vi "RTM - Remove Packet.vi"() -> ()   [LabVIEW 2016, in "UDP-Custom-Device System Explorer.lvlib"]
uses:
  UDP-Custom-Device System Explorer.lvlib
  Shared/Constants.vi
  <vilib>/NI Veristand/Custom Device API/Get Item Property (I32 Array).vi
  <vilib>/NI Veristand/Custom Device API/Get Item Property (String Array).vi
  <vilib>/NI Veristand/Custom Device API/Set Item Property (I32 Array).vi
  <vilib>/NI Veristand/Custom Device API/Set Item Property (String Array).vi
  Shared/UDP-Custom-Device Shared.lvlib
  <vilib>/NI VeriStand/Custom Device API/Custom Device API.lvlib
  <vilib>/NI VeriStand/Custom Device Tools/Custom Device Utility Library/Custom Device Utility Library.lvlib
panel:
  in  "Tag":string
  in  "Node Ptr":u64 format="%.0x"
  out "error out":errorcluster
  in  "error in (no error)":errorcluster
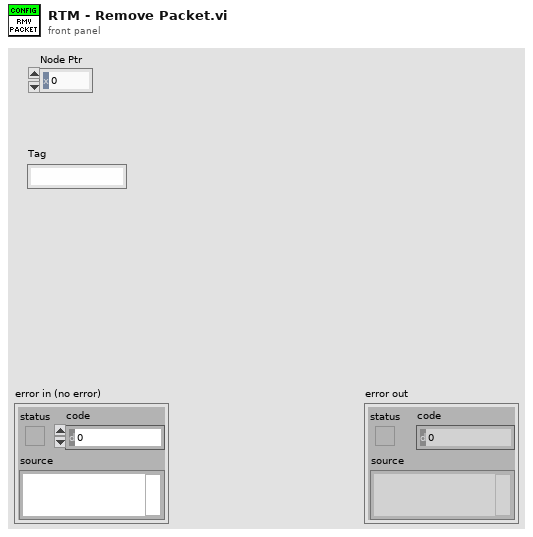
[diagram p1: front panel]
types:
  T1 = typedef "Custom Device API.lvlib/Custom Device Item Ref.ctl" = u64
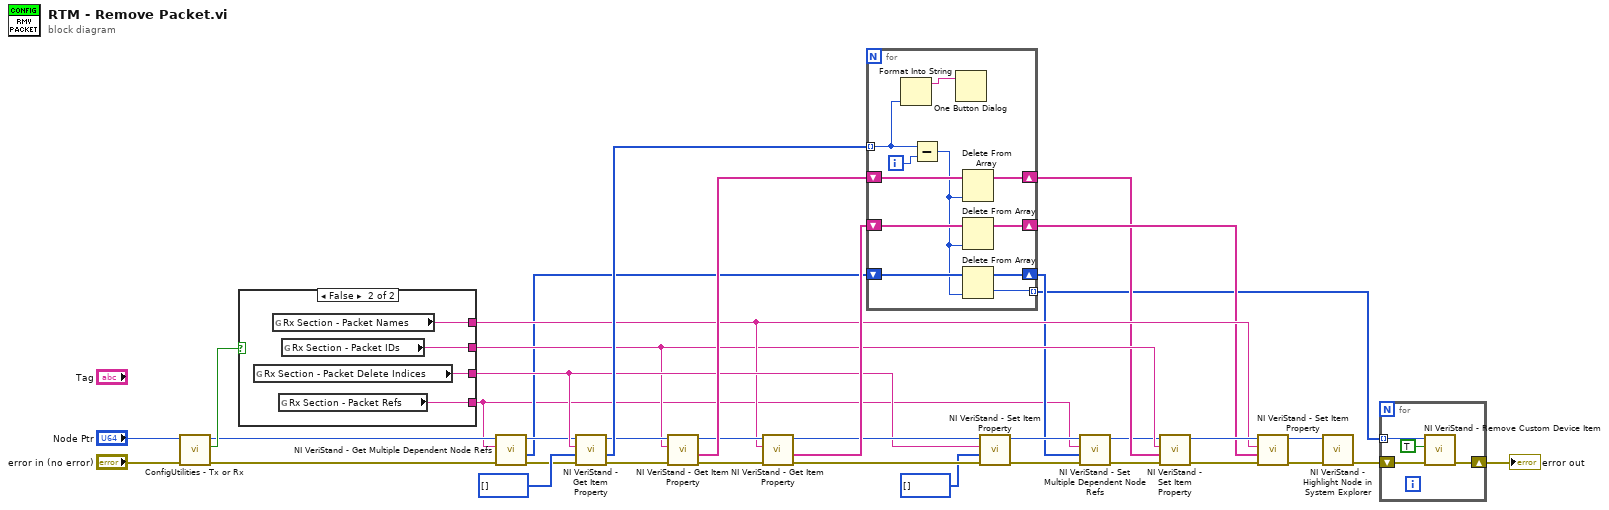
[diagram p0: block diagram]
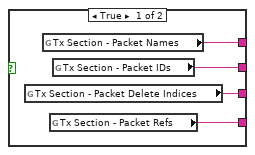
[diagram p2: hidden frame]
diagram:
  n1 = call "ConfigUtilities - Tx or Rx.vi"("error in (no error)"="error in (no error)", "Item Ref in"="Node Ptr") -> ("error out"=w34:errorcluster, "Tx?"=w35:bool, "Item Ref out"=w10:T1)  [unwired: 7 in]
  n2 = case shown="False" w35 {
    tunnel: [w41 w45] -> w19
    tunnel: [w40 w44] -> w18
    tunnel: [w39 w43] -> w23
    tunnel: [w38 w42] -> w3
    frame True {
      n3 = global read "Constants.vi" "Tx Section - Packet Delete Indices"() -> (w39:string)
      n4 = global read "Constants.vi" "Tx Section - Packet Names"() -> (w41:string)
      n5 = global read "Constants.vi" "Tx Section - Packet Refs"() -> (w38:string)
      n6 = global read "Constants.vi" "Tx Section - Packet IDs"() -> (w40:string)
    }
    frame False {
      n7 = global read "Constants.vi" "Rx Section - Packet Delete Indices"() -> (w43:string)
      n8 = global read "Constants.vi" "Rx Section - Packet Names"() -> (w45:string)
      n9 = global read "Constants.vi" "Rx Section - Packet Refs"() -> (w42:string)
      n10 = global read "Constants.vi" "Rx Section - Packet IDs"() -> (w44:string)
    }
  }
  n11 = call <vilib>:"NI VeriStand - Get Multiple Dependent Node Refs.vi"("error in (no error)"=w34, "Base Property Name"=w3, "Item Ref in"=w10) -> ("error out"=w11:errorcluster, "Dependent Node Refs"=w8:T1[], "Item Ref out"=w9:T1)  [unwired: 6 in]
  n12 = call-poly <vilib>:"NI VeriStand - Get Item Property.vi"("error in (no error)"=w11, "Default Value"=i32[] [], "Property Name"=w23, "Item Ref in"=w9) -> ("error out"=w30:errorcluster, "Value"=w31:i32[], "Item Ref out"=w27:T1)  [unwired: 4 in, 1 out]
  n13 = call-poly <vilib>:"NI VeriStand - Get Item Property.vi"("error in (no error)"=w30, "Property Name"=w18, "Item Ref in"=w27) -> ("error out"=w29:errorcluster, "Value"=w32:string[], "Item Ref out"=w28:T1)  [unwired: 5 in, 1 out]
  n14 = call-poly <vilib>:"NI VeriStand - Get Item Property.vi"("error in (no error)"=w29, "Property Name"=w19, "Item Ref in"=w28) -> ("error out"=w24:errorcluster, "Value"=w33:string[], "Item Ref out"=w25:T1)  [unwired: 5 in, 1 out]
  n15 = for {
    shift-right: [w55] -> w16
    shift-left: w32 -> [w56]
    shift-right: [w53] -> w17
    shift-left: w33 -> [w54]
    tunnel: w31 -> [w47] mode=indexing
    shift-right: [w50] -> w4
    shift-left: w8 -> [w52]
    tunnel: [w49] -> w1 mode=indexing
    i -> [w46]
    n16 = Format Into String(w47) -> (resulting string=w48:string)  [unwired: 3 in, 1 out]
    n17 = Subtract(x=w47, y=w46) -> (x-y=w51:i32)
    n18 = One Button Dialog(message=w48) -> ()  [unwired: 1 in, 1 out]
    n19 = Delete From Array(array=w56, index=w51) -> (array with subset deleted=w55:string[])  [unwired: 1 in, 1 out]
    n20 = Delete From Array(array=w54, index=w51) -> (array with subset deleted=w53:string[])  [unwired: 1 in, 1 out]
    n21 = Delete From Array(array=w52, index=w51) -> (deleted portion=w49:T1, array with subset deleted=w50:T1[])  [unwired: 1 in]
  }
  n22 = call-poly <vilib>:"NI VeriStand - Set Item Property.vi"("error in (no error)"=w24, "Value"=i32[] [] ("Default Value"), "Property Name"=w23, "Item Ref in"=w25) -> ("error out"=w21:errorcluster, "Item Ref out"=w6:T1)  [unwired: 5 in, 1 out]
  n23 = call <vilib>:"NI VeriStand - Set Multiple Dependent Node Refs.vi"("error in (no error)"=w21, "Dependent Node Refs"=w4, "Base Property Name"=w3, "Item Ref in"=w6) -> ("error out"=w7:errorcluster, "Item Ref out"=w5:T1)  [unwired: 6 in]
  n24 = call-poly <vilib>:"NI VeriStand - Set Item Property.vi"("error in (no error)"=w7, "Value"=w16, "Property Name"=w18, "Item Ref in"=w5) -> ("error out"=w22:errorcluster, "Item Ref out"=w20:T1)  [unwired: 5 in, 1 out]
  n25 = call-poly <vilib>:"NI VeriStand - Set Item Property.vi"("error in (no error)"=w22, "Value"=w17, "Property Name"=w19, "Item Ref in"=w20) -> ("error out"=w14:errorcluster, "Item Ref out"=w13:T1)  [unwired: 5 in, 1 out]
  n26 = call <vilib>:"NI VeriStand - Highlight Node in System Explorer.vi"("error in (no error)"=w14, "Item Ref in"=w13) -> ("error out"=w12:errorcluster)  [unwired: 8 in, 1 out]
  n27 = for {
    shift-right: [w59] -> w2
    shift-left: w12 -> [w60]
    tunnel: w1 -> [w58] mode=indexing
    n28 = call <vilib>:"NI VeriStand - Remove Custom Device Item.vi"("error in (no error)"=w60, "Force Delete (F)"=TRUE, "Item Ref in"=w58) -> ("error out"=w59:errorcluster)  [unwired: 7 in, 1 out]
  }
  "error out" <- w2
